vi "inertia.vi"(1 "constants":T1, 2 "time elapsed (s)":dbl, 3 "residual":T2, 4 "applied":T3) -> (0 "estimated":T2)   [LabVIEW 2009]
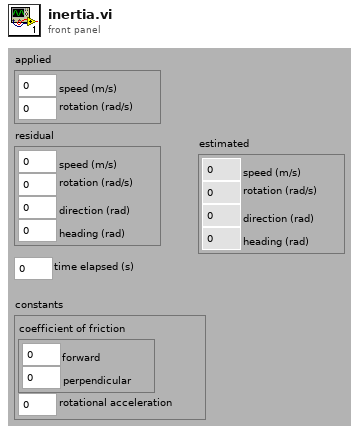
[diagram p1: front panel]
types:
  T1 = cluster{"coefficient of friction":cluster{"forward":dbl, "perpendicular":dbl}, "rotational acceleration":dbl}
  T2 = cluster{"speed (m/s)":dbl, "rotation (rad/s)":dbl, "direction (rad)":dbl, "heading (rad)":dbl}
  T3 = cluster{"speed (m/s)":dbl, "rotation (rad/s)":dbl}
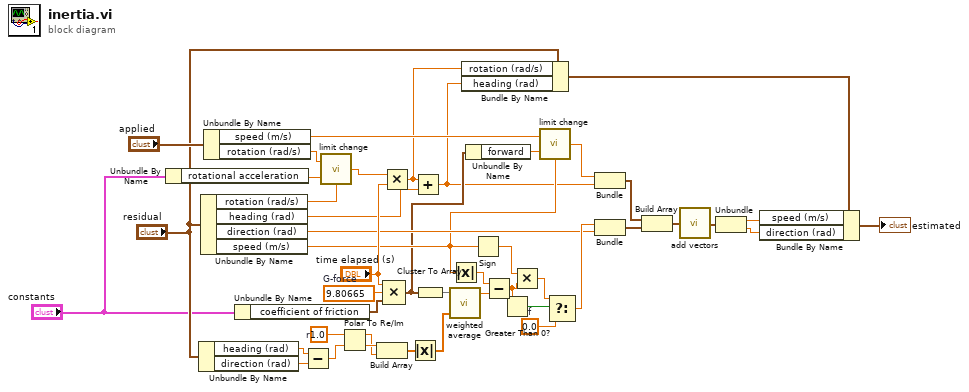
[diagram p0: block diagram]
diagram:
  w25 = 0.0  # f
  w42 = 1.0  # r
  w44 = 9.80665  # G-force
  n1 = Unbundle By Name("constants") -> ("rotational acceleration"=w1:dbl)
  n2 = Unbundle By Name("residual") -> ("heading (rad)"=w40:dbl, "direction (rad)"=w41:dbl)
  n3 = Unbundle By Name("residual") -> ("rotation (rad/s)"=w4:dbl, "heading (rad)"=w32:dbl, "direction (rad)"=w17:dbl, "speed (m/s)"=w13:dbl)
  n4 = Unbundle By Name("applied") -> ("speed (m/s)"=w19:dbl, "rotation (rad/s)"=w3:dbl)
  n5 = Unbundle By Name("constants") -> ("coefficient of friction"=w6:cluster{"forward":dbl, "perpendicular":dbl})
  n6 = Subtract(x=w40, y=w41) -> (x-y=w39:dbl)
  n7 = call "limit change.vi"("previous output"=w4, "max change"=w1, "value"=w3) -> ("output"=w2:dbl)
  n8 = Polar To Re/Im(2:w39, 3:w42) -> (0:w38:dbl, 1:w37:dbl)
  n9 = Build Array(w38, w37) -> (w36:dbl[])
  n10 = Multiply(x=w2, y="time elapsed (s)") -> (x*y=w11:dbl)
  n11 = Compound Arithmetic op=MULTIPLY("time elapsed (s)", w44, w6) -> (w9:cluster{"forward":dbl, "perpendicular":dbl})
  n12 = Absolute Value(x=w36) -> (abs(x)=w35:dbl[])
  n13 = Add(x=w11, y=w32) -> (x+y=w7:dbl)
  n14 = Cluster To Array(cluster=w9) -> (array=w43:dbl[])
  n15 = call "weighted average.vi"("weighting"=w35, "elements"=w43) -> ("average"=w30:dbl)  [unwired: 2 in, 1 out]
  n16 = Absolute Value(x=w13) -> (abs(x)=w31:dbl)
  n17 = Bundle By Name(cluster="residual", "rotation (rad/s)"=w11, "heading (rad)"=w7) -> (w10:T2)
  n18 = Unbundle By Name(w9) -> ("forward"=w8:dbl)
  n19 = Sign(1:w13) -> (0:w27:dbl)
  n20 = Subtract(x=w31, y=w30) -> (x-y=w28:dbl)
  n21 = Greater Than 0?(x=w28) -> (x > 0?=w29:bool)
  n22 = Multiply(x=w27, y=w28) -> (x*y=w26:dbl)
  n23 = call "limit change.vi"("previous output"=w13, "max change"=w8, "value"=w19) -> ("output"=w18:dbl)
  n24 = Select(t=w26, s=w29, f=w25) -> (s? t:f=w20:dbl)
  n25 = Bundle("output"=w18, w7) -> (w15:cluster{"output":dbl, dbl})  [unwired: 1 in]
  n26 = Bundle("f"=w20, "direction (rad)"=w17) -> (w16:cluster{"f":dbl, "direction (rad)":dbl})  [unwired: 1 in]
  n27 = Build Array(w15, w16) -> (w14:cluster{"f":dbl, "direction (rad)":dbl}[])
  n28 = call "add vectors.vi"("vectors"=w14) -> ("vector"=w23:cluster{"length":dbl, "angle":dbl})
  n29 = Unbundle(w23) -> ("length"=w22:dbl, "angle"=w21:dbl)
  n30 = Bundle By Name(cluster=w10, "speed (m/s)"=w22, "direction (rad)"=w21) -> (→"estimated":T2)
